vi "Password.vi"(10 "Log member":enum16{"Admin", "Engineering_Mode", "Operator"}(ring), 11 "Op_name":string) -> (3 "Correct":bool)   [LabVIEW 2024, in "Launcher_DTU.lvlib"]
uses:
  Launcher_DTU.lvlib
  Global 1.vi
panel:
  in  "OK":bool
  in  "Password":string
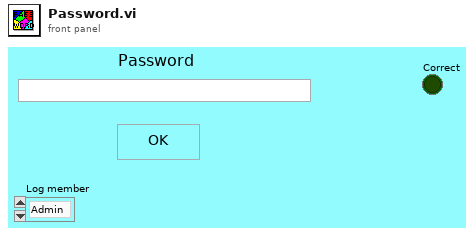
[diagram p1: front panel]
types:
  T1 = cluster{"Password":string, "Op_name":string, "Log member":enum16{"Admin", "Engineering_Mode", "Operator"}}
  T2 = enum16{"Read", "Write", "All_sections", "All_values", "Remove key&section"}
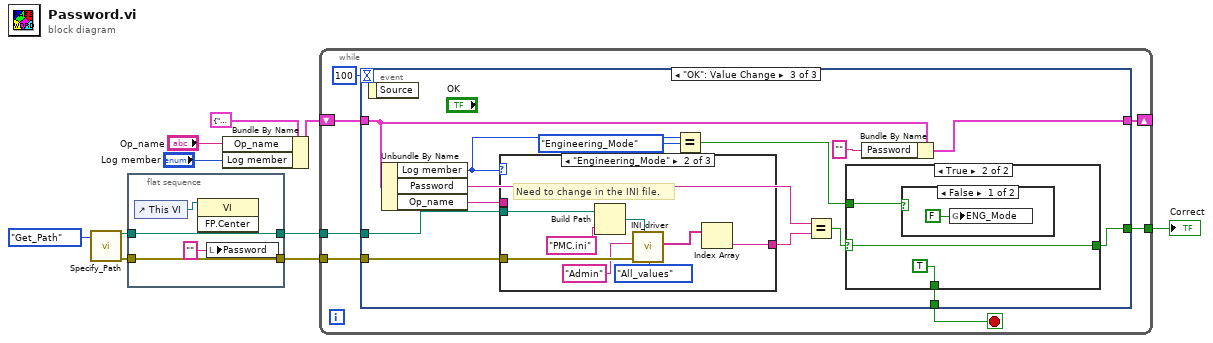
[diagram p0: block diagram]
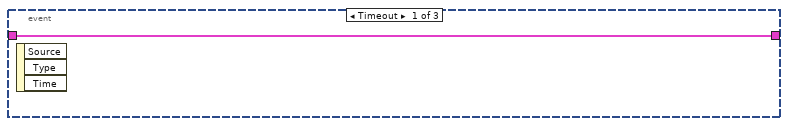
[diagram p2: hidden frame]
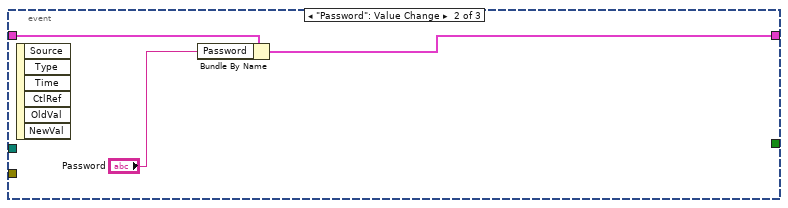
[diagram p3: hidden frame]
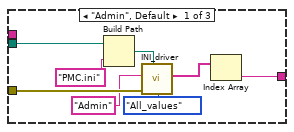
[diagram p4: hidden frame]
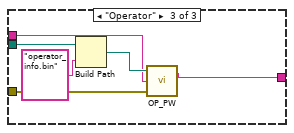
[diagram p5: hidden frame]
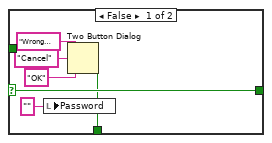
[diagram p6: hidden frame]
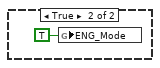
[diagram p7: hidden frame]
diagram:
  n1 = call "Specify_Path.vi"("Path_Enum"=enum16{"Find_Path", "Get_Path"}."Get_Path") -> ("Configurations"=w7:path, "error out"=w6:errorcluster)  [unwired: 7 in, 6 out]
  n2 = flat-sequence {
    tunnel: w7 -> [w13]
    tunnel: w6 -> [w14]
    tunnel: [w14] -> w4
    tunnel: [w13] -> w5
    frame #0 {
      n3 = control-ref of="This VI"() -> (w11:refnum<vi>)
      n4 = invoke class="VI" method="FP.Center"(reference=w11) -> ()  [unwired: 2 in, 3 out]
      n5 = local write "Password"("" ("Password")) -> ()
    }
  }
  n6 = Bundle By Name(cluster=T1 {"Password"="", "Op_name"="", "Log member"=enum."Admin"}, "Op_name"="Op_name", "Log member"="Log member") -> (w3:T1)
  n7 = while {
    tunnel: w4 -> [w20]
    tunnel: w5 -> [w19]
    shift-right: [w17] -> _
    shift-left: w3 -> [w18]
    tunnel: [w15] -> w8
    stop <- w16 stop-if-true
    n8 = event shown="[2] \"OK\": Value Change" {
      selector: _ -> [_ _ _]
      dyn-events: _ -> [_ _ _]
      timeout: 100 -> [_ _ _]
      tunnel: w20 -> [_ _ w36]
      tunnel: w19 -> [_ _ w35]
      tunnel: w18 -> [w22 w25 w39]
      tunnel: [w22 w24 w38] -> w17
      tunnel: [_ _ w31] -> w16
      tunnel: [_ _ w30] -> w15
      event Timeout {
        n9 = event-data() -> ()  [unwired: 1 in, 3 out]
      }
      event "Password": Value Change {
        n10 = event-data() -> ()  [unwired: 1 in, 6 out]
        n11 = Bundle By Name(cluster=w25, "Password"="Password") -> (w24:T1)
      }
      event "OK": Value Change {
        n12 = event-data() -> ()  [unwired: 1 in, 1 out]
        n13 = Unbundle By Name(w39) -> ("Log member"=w28:enum16{"Admin", "Engineering_Mode", "Operator"}, "Password"=w33:string, "Op_name"=w29:string)
        n14 = case shown="\"Engineering_Mode\"" w28 {
          tunnel: w36 -> [w47 w55 w58]
          tunnel: w35 -> [w46 w54 w61]
          tunnel: [w40 w48 w57] -> w34
          tunnel: w29 -> [_ _ w56]
          frame "Admin", Default {
            n15 = Build Path(base path=w46, name or relative path="PMC.ini") -> (appended path=w44:path)
            n16 = call "INI_driver.vi"("Enum"=T2."All_values", "instrument file path"=w44, "error in (no error)"=w47, "Section"="Admin") -> ("Values out"=w41:string[])  [unwired: 4 in, 3 out]
            n17 = Index Array(array=w41) -> (element=w40:string)  [unwired: 1 in]
          }
          frame "Engineering_Mode" {
            # "Need to change in the INI file."
            n18 = Build Path(base path=w54, name or relative path="PMC.ini") -> (appended path=w52:path)
            n19 = call "INI_driver.vi"("Enum"=T2."All_values", "instrument file path"=w52, "error in (no error)"=w55, "Section"="Admin") -> ("Values out"=w49:string[])  [unwired: 4 in, 3 out]
            n20 = Index Array(array=w49) -> (element=w48:string)  [unwired: 1 in]
          }
          frame "Operator" {
            n21 = Build Path(base path=w61, name or relative path="operator_info.bin") -> (appended path=w59:path)
            n22 = call "OP_PW.vi"("error in"=w58, "Op_name"=w56, "Path"=w59) -> ("Password"=w57:string)  [unwired: 1 out]
          }
        }
        n23 = Equal?(x=w28, y=enum16{"Admin", "Engineering_Mode", "Operator"}."Engineering_Mode") -> (x = y?=w26:bool)
        n24 = Equal?(x=w33, y=w34) -> (x = y?=w32:bool)
        n25 = case shown="True" w32 {
          selector: w32 -> [w66 w69]
          tunnel: [w63 TRUE] -> w31
          tunnel: [w66 w69] -> w30
          tunnel: w26 -> [_ w68]
          frame False {
            n26 = local write "Password"("" ("Password")) -> ()
            n27 = Two Button Dialog(message="Wrong Password !!!", 1:"OK" ("F button name (\"Cancel\")"), 2:"Cancel" ("T button name (\"OK\")")) -> (T button?=w63:bool)
          }
          frame True {
            n28 = case shown="False" w68 {
              frame False {
                n29 = global write "Global 1.vi" "ENG_Mode"(FALSE ("ENG_Mode")) -> ()
              }
              frame True {
                n30 = global write "Global 1.vi" "ENG_Mode"(TRUE ("ENG_Mode")) -> ()
              }
            }
          }
        }
        n31 = Bundle By Name(cluster=w39, "Password"="") -> (w38:T1)
      }
    }
  }
  "Correct" <- w8
